vi "Build Description String.vi"(8 "error in (no error)":errorcluster, 11 "Numeric Assertion in":refnum<class "Numeric Assertion.lvclass">) -> (0 "error out":errorcluster, 2 "Description":string, 3 "Numeric Assertion out":refnum<class "Numeric Assertion.lvclass">)   [LabVIEW 2020, in "MacroAssert.lvlib" / "Numeric Assertion.lvclass"]
doc: "Builds a string to describe what <B>Step</B> does."
uses:
  Numeric Assertion.lvclass
  C:/Users/acasalen/Documents/LabVIEW Data/Projects/MacroAssert/source/Classes/Assertion Step/Assertion Step.lvclass
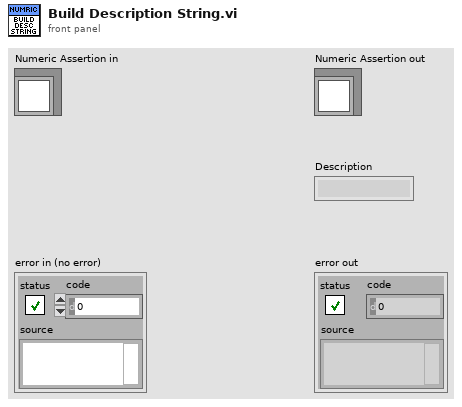
[diagram p1: front panel]
types:
  T1 = enum8{"Enabled", "Disabled", "Disabled and Grayed Out"}
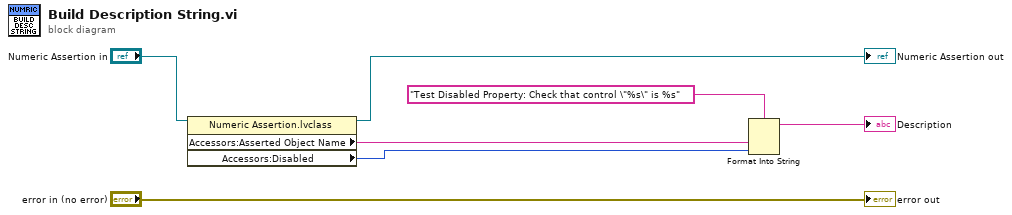
[diagram p0: block diagram]
diagram:
  n1 = property class="Numeric Assertion.lvclass"(reference="Numeric Assertion in") -> (reference out=→"Numeric Assertion out":refnum<class "Numeric Assertion.lvclass">, "Accessors:Asserted Object Name"=w5:string, "Accessors:Disabled"=w3:T1)  [unwired: 1 in, 1 out]
  n2 = Format Into String(format string="Test Disabled Property: Check that control \"%s\" is %s", w5, w3) -> (resulting string=→"Description":string)  [unwired: 2 in, 1 out]
  "error out" <- "error in (no error)"
